vi "delete EIP tag.vi"(8 "error in":errorcluster, 9 "Tag Name":string, 10 "Network Path":string, 11 "EIP Tags configuration in":refnum<class "EIP Tags Configuration.lvclass">) -> (0 "error out":errorcluster, 2 "removed channels":refnum<class "EIP Tags Channel.lvclass">[](array[class]), 3 "EIP Tags configuration out":refnum<class "EIP Tags Configuration.lvclass">)   [LabVIEW 2013, in "EIP Tags Configuration.lvclass"]
uses:
  EIP Tags Configuration.lvclass
  channel/EIP Tags Channel.lvclass
  EIP Tags Configuration.lvclass/EIP Tags Configuration.ctl
  channel/EIP Tags Channel.lvclass/EIP Tags Channel.ctl
  channel/Read EIP Tag UUID.vi
  <vilib>/NI/Configuration Framework/NISE_CEF_TreeControl.lvlib
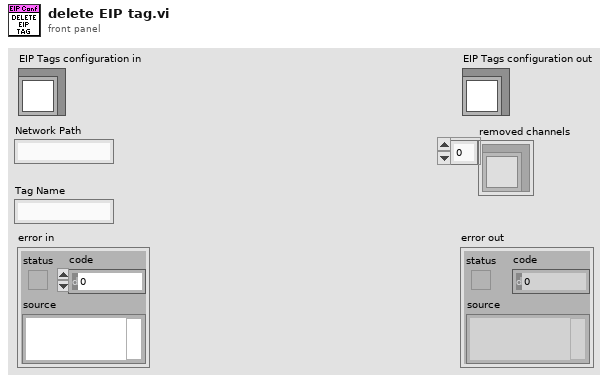
[diagram p1: front panel]
types:
  T1 = typedef "EIP Tags Configuration.lvclass/eip tag definition.ctl" = cluster{"eip tag types":T2, "unique tag name":string, "Number of Elements":u32}
  T2 = typedef "EIP Tags Configuration.lvclass/eip tag types.ctl" = enum16{"SINT", "INT", "DINT", "REAL", "BOOL", "STRING"}
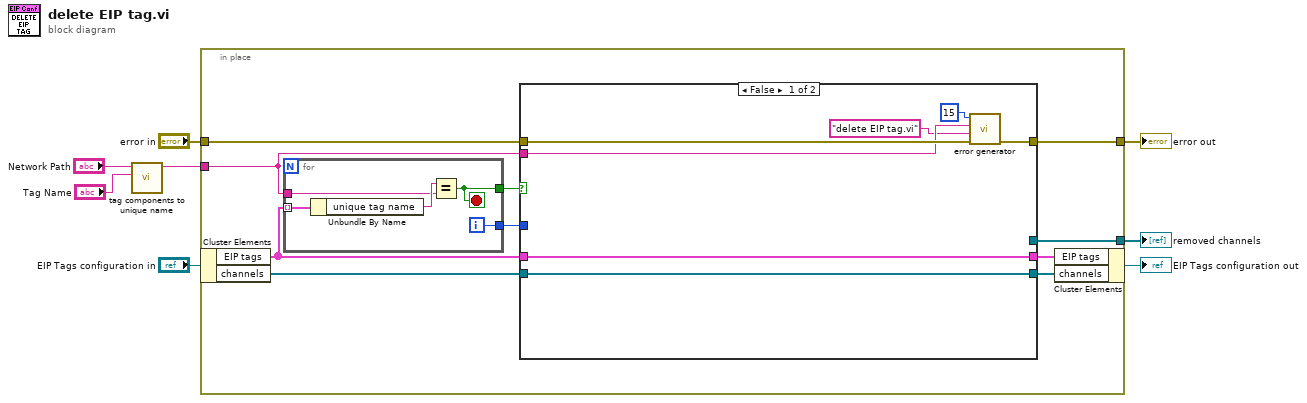
[diagram p0: block diagram]
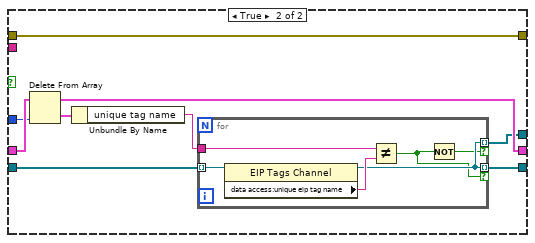
[diagram p2: hidden frame]
diagram:
  n1 = call "tag components to unique name.vi"("Tag Name"="Tag Name", "Network Path"="Network Path") -> ("unique name"=w3:string)  [unwired: 9 in]
  n2 = in-place {
    in-place-border: "error in" -> [w16]
    in-place-border: w3 -> [w13]
    in-place-border: [w17] -> w2
    in-place-border: [w9] -> w1
    n3 = in-place-cluster #1("EIP Tags configuration in") -> ("EIP tags"=w14:T1[], "channels"=w11:refnum<class "EIP Tags Channel.lvclass">[])
    n4 = for {
      tunnel: w14 -> [w45] mode=indexing
      tunnel: w13 -> [w43]
      tunnel: [w42] -> w18
      tunnel: [w41] -> w12
      i -> [w41]
      stop <- w42 stop-if-true
      n5 = Unbundle By Name(w45) -> ("unique tag name"=w44:string)
      n6 = Equal?(x=w44, y=w43) -> (x = y?=w42:bool)
    }
    n7 = case shown="False" w18 {
      tunnel: [w25 w34] -> w17
      tunnel: w16 -> [w24 w34]
      tunnel: [w22 w32] -> w15
      tunnel: w14 -> [w22 w33]
      tunnel: w13 -> [w21 _]
      tunnel: w12 -> [_ w31]
      tunnel: w11 -> [w19 w30]
      tunnel: [w19 w27] -> w10
      tunnel: [_ w26] -> w9
      frame False {
        n8 = call <vilib>:"error generator.vi"("error in"=w24, "source"="delete EIP tag.vi", "append error message"=w21, "error code (0)"=15) -> ("error out"=w25:errorcluster)  [unwired: 5 in]
      }
      frame True {
        n9 = Delete From Array(array=w33, index=w31) -> (deleted portion=w29:T1, array with subset deleted=w32:T1[])  [unwired: 1 in]
        n10 = Unbundle By Name(w29) -> ("unique tag name"=w28:string)
        n11 = for {
          tunnel: w30 -> [w40] mode=indexing
          tunnel: w28 -> [w39]
          tunnel: [w37] -> w27 mode=indexing if=w35
          tunnel: [w37] -> w26 mode=indexing if=w36
          n12 = property class="EIP Tags Channel"(reference=w40) -> (reference out=w37:refnum<class "EIP Tags Channel.lvclass">, "data access:unique eip tag name"=w38:string)  [unwired: 1 in, 1 out]
          n13 = Not Equal?(x=w39, y=w38) -> (x != y?=w35:bool)
          n14 = Not(x=w35) -> (.not. x?=w36:bool)
        }
      }
    }
    n15 = in-place-cluster #1("EIP tags"=w15, "channels"=w10) -> (→"EIP Tags configuration out":refnum<class "EIP Tags Configuration.lvclass">)
  }
  "error out" <- w2
  "removed channels" <- w1
